vi "FGV AutoKAL Daten.vi"(6 "Aktionen":T2, 11 "Aufschaltzeiten":T1) -> (3 "Aufschaltzeiten":T1)   [LabVIEW 2020, in "Auto Kalibrieren.lvlib"]
uses:
  Auto Kalibrieren.lvlib
  Aktionen FGV AutoKAL Daten.ctl
  Auschaltzeiten Null Endpunktgase.ctl
  Allgemein/allgemeine Sub-VIs.lvlib
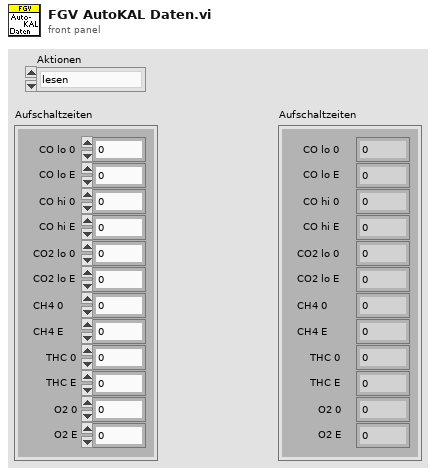
[diagram p1: front panel]
types:
  T1 = typedef "Auto Kalibrieren.lvlib/Auschaltzeiten Null Endpunktgase.ctl" = cluster{"CO lo 0":sgl, "CO lo E":sgl, "CO hi 0":sgl, "CO hi E":sgl, "CO2 lo 0":sgl, "CO2 lo E":sgl, "CH4 0":sgl, "CH4 E":sgl, "THC 0":sgl, "THC E":sgl, "O2 0":sgl, "O2 E":sgl}
  T2 = typedef "Auto Kalibrieren.lvlib/Aktionen FGV AutoKAL Daten.ctl" = enum16{"lesen", "laden", "speichern", "Aufschaltzeit"}
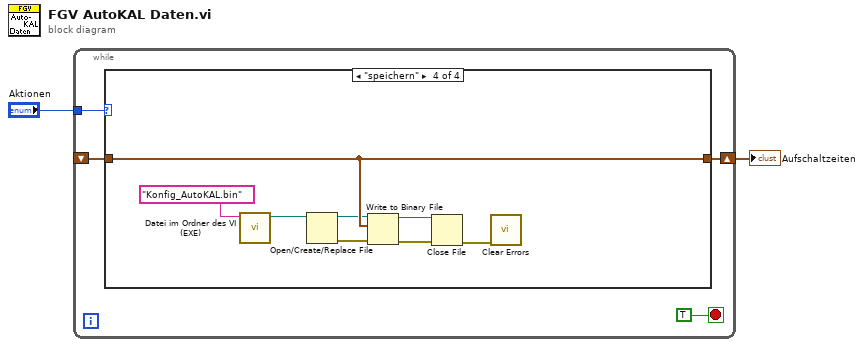
[diagram p0: block diagram]
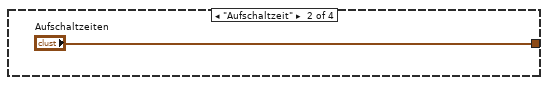
[diagram p3: hidden frame]
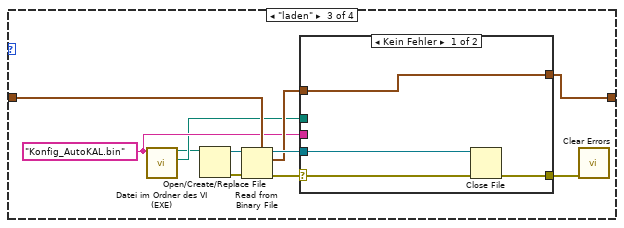
[diagram p4: hidden frame]
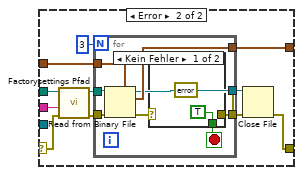
[diagram p5: hidden frame]
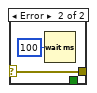
[diagram p6: hidden frame]
diagram:
  n1 = while {
    tunnel: "Aktionen" -> [w6]
    shift-right: [w3] -> w1
    shift-left: _ -> [w4]
    stop <- TRUE stop-if-true
    n2 = case shown="\"speichern\"" w6 {
      tunnel: w4 -> [w7 _ w19 w53]
      tunnel: [w7 "Aufschaltzeiten" w13 w53] -> w3
      frame "lesen", Default {
      }
      frame "Aufschaltzeit" {
      }
      frame "laden" {
        w15 = "Konfig_AutoKAL.bin" ("Dateiname")
        n3 = call "Datei im Ordner des VI (EXE).vi"("Dateiname"=w15) -> ("Ordner des Haupt-VIs"=w14:path, "Dateipfad im Ordner des Haupt-VIs"=w9:path)  [unwired: 8 in, 1 out]
        n4 = Open/Create/Replace File(file path (use dialog)=w9) -> (refnum out=w10:refnum<file>, error out=w11:errorcluster)  [unwired: 5 in, 1 out]
        n5 = Read from Binary File(5:w19, 8:w11, 11:w10) -> (0:w18:errorcluster, 2:w16:T1, 3:w17:refnum<file>)  [unwired: 4 out]
        n6 = case shown="Kein Fehler" w18 {
          selector: w18 -> [w22 w26]
          tunnel: w14 -> [_ w27]
          tunnel: w16 -> [w23 w25]
          tunnel: [w23 w33] -> w13
          tunnel: [w20 w31] -> w12
          tunnel: w17 -> [w21 _]
          tunnel: w15 -> [_ w24]
          frame No Error {
            n7 = Close File(refnum=w21, error in=w22) -> (error out=w20:errorcluster)  [unwired: 1 out]
          }
          frame Error {
            n8 = call "Factorysettings Pfad.vi"("error in (no error)"=w26, "Dateiname"=w24, "Ordner des Haupt-VIs"=w27) -> ("error out"=w28:errorcluster, "Pfad Factorysettings"=w29:path)  [unwired: 7 in]
            n9 = for {
              N: 3 -> [_]
              tunnel: w28 -> [w40]
              tunnel: w29 -> [w39]
              tunnel: [w38] -> w33
              tunnel: [w37] -> w32
              tunnel: [w36] -> w30
              tunnel: w25 -> [w35]
              stop <- w41 stop-if-true
              n10 = Read from Binary File(5:w35, 8:w40, 11:w39) -> (0:w42:errorcluster, 2:w38:T1, 3:w36:refnum<file>)  [unwired: 3 in, 1 out]
              n11 = case shown="Kein Fehler" w42 {
                selector: w42 -> [_ w45]
                tunnel: [TRUE _] -> w41
                tunnel: [errorcluster {"status"=FALSE, "code"=0, "source"=""} ("error IO") w45] -> w37
                frame No Error {
                }
                frame Error {
                  n12 = Wait (ms)(milliseconds to wait=u32 100 ("Zu wartende ms")) -> ()  [unwired: 1 out]
                }
              }
            }
            n13 = Close File(refnum=w30, error in=w32) -> (error out=w31:errorcluster)  [unwired: 1 out]
          }
        }
        n14 = call <vilib>:"Clear Errors.vi"("error in (no error)"=w12) -> ()  [unwired: 5 in, 2 out]
      }
      frame "speichern" {
        n15 = call "Datei im Ordner des VI (EXE).vi"("Dateiname"="Konfig_AutoKAL.bin") -> ("Dateipfad im Ordner des Haupt-VIs"=w52:path)  [unwired: 8 in, 2 out]
        n16 = Open/Create/Replace File(file path (use dialog)=w52) -> (refnum out=w50:refnum<file>, error out=w51:errorcluster)  [unwired: 5 in, 1 out]
        n17 = Write to Binary File(file (use dialog)=w50, data=w53, error in=w51) -> (refnum out=w49:refnum<file>, error out=w48:errorcluster)  [unwired: 1 in, 3 out]
        n18 = Close File(refnum=w49, error in=w48) -> (error out=w47:errorcluster)  [unwired: 1 out]
        n19 = call <vilib>:"Clear Errors.vi"("error in (no error)"=w47) -> ()  [unwired: 5 in, 2 out]
      }
    }
  }
  "Aufschaltzeiten" <- w1
